vi "Teleop.vi"(9 "Match Info":T1={"Autonomous Elapsed Seconds"=0.0, "TeleOp Elapsed Seconds"=0.0, "Disabled Elapsed Seconds"=0.0, "Visited Autonomous"=FALSE, "Visited TeleOp"=FALSE, "Visited Disabled"=FALSE, "Autonomous Settings"={"Autonomous Style"=enum."Independent", "VI Refnum"=refnum}}, 11 "Call Context":T2) -> ()   [LabVIEW 2014]
doc: "This VI is called for each TeleOp packet received from the DS where the robot is not disabled. It is often used to read from the joysticks and update I/O or to update setpoints for timed control loops. It should complete and return within 20 milliseconds or it may miss DS packets."
uses:
  <vilib>/Rock Robotics/WPI/DriverStation/WPI_DriverStationDerivedRobotMode.ctl
  <vilib>/Rock Robotics/WPI/DriverStation/WPI_DriverStationMatch Info.ctl
  <vilib>/Rock Robotics/WPI/RobotDrive/WPI_RobotDriveGetSetRefNum.vi
  <vilib>/Rock Robotics/WPI/Joystick/WPI_JoystickGetSetRefNum.vi
  <vilib>/Rock Robotics/Network Tables/SD Write Boolean Array.vi
  <vilib>/Rock Robotics/Network Tables/SD Write Numeric Array.vi
  <vilib>/Rock Robotics/WPI/RobotDrive/WPI_RobotDriveMecanumDrive_Cartesian.vi
  <vilib>/Rock Robotics/Network Tables/SD Write Boolean.vi
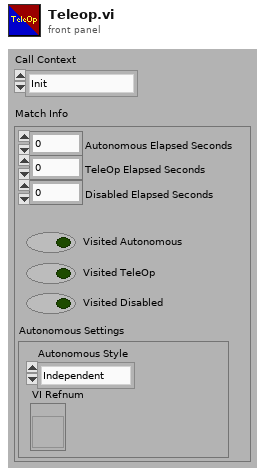
[diagram p1: front panel]
types:
  T1 = typedef "WPI_DriverStationMatch Info.ctl" = cluster{"Autonomous Elapsed Seconds":dbl, "TeleOp Elapsed Seconds":dbl, "Disabled Elapsed Seconds":dbl, "Visited Autonomous":bool, "Visited TeleOp":bool, "Visited Disabled":bool, "Autonomous Settings":cluster{"Autonomous Style":enum16{"Iterative", "Independent"}, "VI Refnum":refnum<vi>}}
  T2 = typedef "WPI_DriverStationDerivedRobotMode.ctl" = enum16{"Init", "Execute", "Stop"}
  T3 = typedef "WPI_RobotDriveDevRef.ctl" = cluster{"DevStatus":errorcluster, "Motors[]":T4[], "Square Inputs":bool, "Max Output":dbl}
  T4 = typedef "WPI_MotorControlDeviceRef.ctl" = cluster{"DeviceStatus":errorcluster, "Type":T5, "PWM":cluster{"Controller":T6, "PWM Channel":T7, "DeadBand":T8}, "CAN":cluster{"Device Number":u8, "Control Mode":T9, "Semaphore":T10, "Max Vout":dbl, "TalonSRX Control Mode":T11}, "Invert":bool, "TransformRef":T12, "InvTransformRef":T12}
  T5 = typedef "WPI_MotorControlType.ctl" = enum16{"PWM", "CAN", "CANTalonSRX"}
  T6 = typedef "FPGA_TypedefDigitalModule.ctl" = enum16{"Controller 1"}
  T7 = typedef "FPGA_DIOPWMChannel.ctl" = enum8{"PWM 0", "PWM 1", "PWM 2", "PWM 3", "PWM 4", "PWM 5", "PWM 6", "PWM 7", "PWM 8", "PWM 9", "PWM MXP 0", "PWM MXP 1", "PWM MXP 2", "PWM MXP 3", "PWM MXP 4", "PWM MXP 5", "PWM MXP 6", "PWM MXP 7", "PWM MXP 8", "PWM MXP 9", "Invalid"}
  T8 = typedef "WPI_PWMDeadband.ctl" = cluster{"Name":string, "maxPositivePwm":i32, "minPositivePwm":i32, "centerPwm":i32, "maxNegativePwm":i32, "minNegativePwm":i32, "angularRange":u16}
  T9 = typedef "WPI_CANJaguar_ControlMode.ctl" = enum8{"Percent VBus", "Current", "Speed", "Position", "Voltage"}
  T10 = typedef "Semaphore RefNum" = refnum<k1>
  T11 = typedef "WPI_CANTalonSRX_APIControlMode.ctl" = enum8{"Percent VBus", "Speed", "Position", "Slave", "Unchanged / Invalid"}
  T12 = typedef "WPI_PWMTransform_ConPane.ctl" = refnum<vi>
  T13 = typedef "WPI_JoystickDevRef.ctl" = cluster{"Device":T14}
  T14 = typedef "WPI_JoystickDeviceEnum.ctl" = enum16{"USB 0", "USB 1", "USB 2", "USB 3", "USB 4", "USB 5"}
  T15 = typedef "WPI_DigitalInputDevRef.ctl" = cluster{"DevStatus":errorcluster, "DIO Channel":T16, "Controller":T6}
  T16 = typedef "FPGA_DIOChannel.ctl" = enum8{"DIO 0", "DIO 1", "DIO 2", "DIO 3", "DIO 4", "DIO 5", "DIO 6", "DIO 7", "DIO 8", "DIO 9", "DIO MXP 0", "DIO MXP 1", "DIO MXP 2", "DIO MXP 3", "DIO MXP 4", "DIO MXP 5", "DIO MXP 6", "DIO MXP 7", "DIO MXP 8", "DIO MXP 9", "DIO MXP 10", "DIO MXP 11", "DIO MXP 12", "DIO MXP 13", "DIO MXP 14", "DIO MXP 15", "Invalid"}
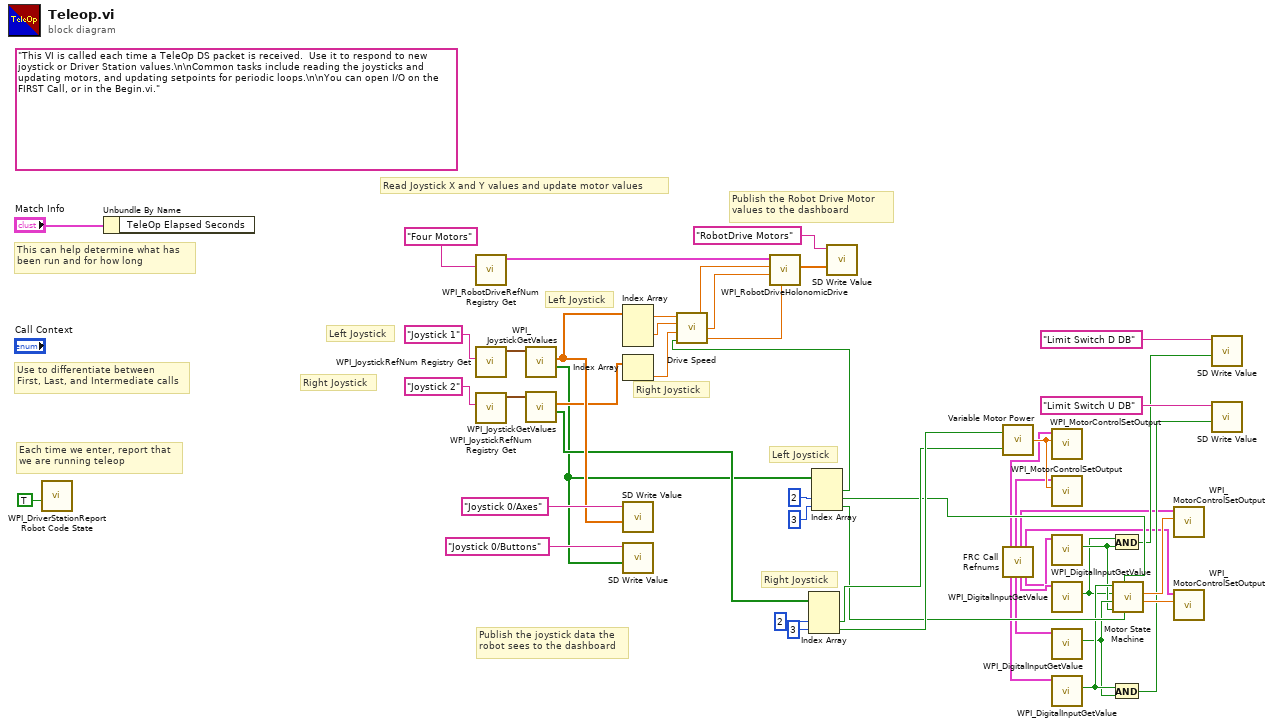
[diagram p0: block diagram]
diagram:
  (unwired) "This VI is called each time a TeleOp DS packet is received.  Use it to respond to new joystick or Driver Station values.\n\nCommon tasks include reading the joysticks and updating motors, and updating setpoints for periodic loops.\n\nYou can open I/O on the FIRST Call, or in the Begin.vi."
  # "Right Joystick"
  # "Left Joystick"
  # "Left Joystick"
  # "Right Joystick"
  # "Left Joystick"
  # "Right Joystick"
  # "Publish the Robot Drive Motor\nvalues to the dashboard"
  # "Publish the joystick data the\nrobot sees to the dashboard"
  # "Each time we enter, report that\nwe are running teleop"
  # "Use to differentiate between\nFirst, Last, and Intermediate calls"
  # "This can help determine what has\nbeen run and for how long"
  # "Read Joystick X and Y values and update motor values"
  n1 = call <vilib>:"WPI_DriverStationReport Robot Code State.vi"("TeleOp"=TRUE ("Autonomous")) -> ()  [unwired: 10 in, 1 out]
  n2 = Unbundle By Name("Match Info") -> ()  [unwired: 1 out]
  n3 = call <vilib>:"WPI_RobotDriveRefNum Registry Get.vi"("refnum name"="Four Motors") -> ("RobotDriveDevRef"=w48:T3)  [unwired: 1 in, 9 out]
  n4 = call <vilib>:"WPI_JoystickRefNum Registry Get.vi"("refnum name"="Joystick 1") -> ("JoystickDevRef"=w46:T13)  [unwired: 1 in, 9 out]
  n5 = call <vilib>:"WPI_JoystickRefNum Registry Get.vi"("refnum name"="Joystick 2") -> ("JoystickDevRef"=w38:T13)  [unwired: 1 in, 9 out]
  n6 = call <vilib>:"WPI_JoystickGetValues.vi"("JoystickDevRef"=w46) -> ("Buttons"=w35:bool[], "Axes"=w40:dbl[])  [unwired: 6 in, 3 out]
  n7 = call <vilib>:"WPI_JoystickGetValues.vi"("JoystickDevRef"=w38) -> ("Buttons"=w36:bool[], "Axes"=w37:dbl[])  [unwired: 6 in, 3 out]
  n8 = Index Array(array=w40) -> (element #1=w31:dbl, element #2=w26:dbl)  [unwired: 3 in, 1 out]
  n9 = Index Array(array=w37) -> (element=w30:dbl)  [unwired: 1 in]
  n10 = call-poly <vilib>:"SD Write Value.vi"("Numeric Array"=w40, "Name"="Joystick 0/Axes") -> ()  [unwired: 8 in, 2 out]
  n11 = call-poly <vilib>:"SD Write Value.vi"("Boolean Array"=w35, "Name"="Joystick 0/Buttons") -> ()  [unwired: 8 in, 2 out]
  n12 = Index Array(array=w36, index #2=2 ("index"), index #3=3 ("index")) -> (element #2=w23:bool, element #3=w24:bool)  [unwired: 1 in, 1 out]
  n13 = Index Array(array=w35, index #2=2 ("index"), index #3=3 ("index")) -> (element #1=w29:bool, element #2=w18:bool, element #3=w17:bool)  [unwired: 1 in]
  n14 = call "Drive Speed.vi"("X"=w31, "Y"=w26, "Rotation"=w30, "Enabled?"=w29) -> ("X Out"=w28:dbl, "Y Out"=w25:dbl, "Rotation Out"=w27:dbl)  [unwired: 2 in]
  n15 = call-poly <vilib>:"WPI_RobotDriveHolonomicDrive.vi"("Rotation"=w27, "Y"=w25, "X"=w28, "RobotDriveDevRef"=w48) -> ("Motor Values"=w41:dbl[])  [unwired: 5 in, 2 out]
  n16 = call-poly <vilib>:"SD Write Value.vi"("Numeric Array"=w41, "Name"="RobotDrive Motors") -> ()  [unwired: 8 in, 2 out]
  n17 = call "Variable Motor Power.vi"("Power Off"=w23, "Power On"=w24) -> ("Motor(s) Out"=w22:dbl)
  n18 = call "FRC Call Refnums.vi"() -> ("End Defector 1"=w4:T4, "Limit Switch LU"=w8:T15, "End Defector 2"=w3:T4, "Limit Switch LD"=w7:T15, "Lifter L"=w2:T4, "Limit Switch RU"=w6:T15, "Lifter D"=w1:T4, "Limit Switch RD"=w5:T15)  [unwired: 11 in, 1 out]
  n19 = call <vilib>:"WPI_MotorControlSetOutput.vi"("Output"=w22, "MotorControlDevRef"=w4) -> ()  [unwired: 7 in, 3 out]
  n20 = call <vilib>:"WPI_MotorControlSetOutput.vi"("Output"=w22, "MotorControlDevRef"=w3) -> ()  [unwired: 7 in, 3 out]
  n21 = call <vilib>:"WPI_DigitalInputGetValue.vi"("DigitalInputDevRef"=w5) -> ("Value"=w10:bool)  [unwired: 8 in, 2 out]
  n22 = call <vilib>:"WPI_DigitalInputGetValue.vi"("DigitalInputDevRef"=w6) -> ("Value"=w9:bool)  [unwired: 8 in, 2 out]
  n23 = call <vilib>:"WPI_DigitalInputGetValue.vi"("DigitalInputDevRef"=w7) -> ("Value"=w11:bool)  [unwired: 8 in, 2 out]
  n24 = call <vilib>:"WPI_DigitalInputGetValue.vi"("DigitalInputDevRef"=w8) -> ("Value"=w12:bool)  [unwired: 8 in, 2 out]
  n25 = And(x=w9, y=w10) -> (x .and. y?=w13:bool)
  n26 = And(x=w12, y=w11) -> (x .and. y?=w14:bool)
  n27 = call "Motor State Machine.vi"("Button D"=w17, "Button U"=w18, "Limit RD"=w10, "Limit RU"=w11, "Limit LD"=w9, "Limit LU"=w12) -> ("Motor Out R"=w20:dbl, "Motor Out L"=w21:dbl)  [unwired: 4 in]
  n28 = call <vilib>:"WPI_MotorControlSetOutput.vi"("Output"=w21, "MotorControlDevRef"=w2) -> ()  [unwired: 7 in, 3 out]
  n29 = call <vilib>:"WPI_MotorControlSetOutput.vi"("Output"=w20, "MotorControlDevRef"=w1) -> ()  [unwired: 7 in, 3 out]
  n30 = call-poly <vilib>:"SD Write Value.vi"("Boolean"=w13, "Name"="Limit Switch D DB" ("refnum name")) -> ()  [unwired: 8 in, 2 out]
  n31 = call-poly <vilib>:"SD Write Value.vi"("Boolean"=w14, "Name"="Limit Switch U DB" ("refnum name")) -> ()  [unwired: 8 in, 2 out]
